vi "qHDI.vi"(0 "System no.":i32=1 min=1 max=4 step=1, 5 "error in":errorcluster) -> (14 "Diagnosis help string":string, 19 "error out":errorcluster)   [LabVIEW 2020]
doc: "Returns help on diagnosis information, received with DIA?. \n\nC-867, C-887, C-891:"
panel:
  # "Get  help on diagnosis information, received with DIA?."
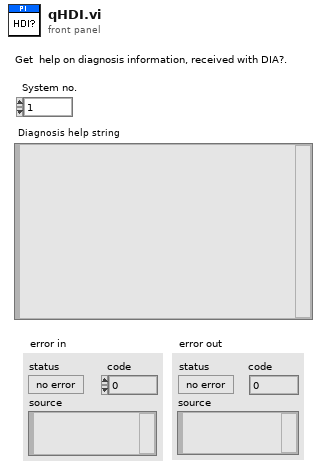
[diagram p1: front panel]
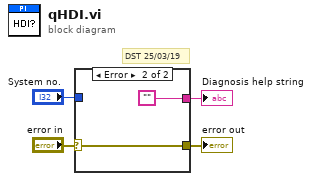
[diagram p0: block diagram]
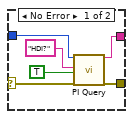
[diagram p2: hidden frame]
diagram:
  # "DST 25/03/19"
  n1 = case shown="Error" "error in" {
    selector: "error in" -> [w5 w12]
    tunnel: "System no." -> [w8 _]
    tunnel: [w7 ""] -> w3
    tunnel: [w6 w12] -> w2
    frame No Error {
      n2 = call "PI Query.vi"("System no."=w8, "String to send"="HDI?" ("String to Send"), "Attach termination char.?"=TRUE ("Attach Linefeed?"), "error in"=w5) -> ("String read"=w7:string, "error out"=w6:errorcluster)  [unwired: 3 in, 11 out]
    }
    frame Error {
    }
  }
  "Diagnosis help string" <- w3
  "error out" <- w2
